vi "RSZVB Set Permanent Signal Generator State.vi"(6 "Generator Number (1)":i32=1, 7 "State (F: Off)":bool, 8 "error in (no error)":errorcluster {"code" format="%.0x"}, 9 "Port (1)":i32=1, 10 "Channel (1)":i32=1, 11 "VISA session":refnum<visa-resource-name>) -> (0 "error out":errorcluster {"code" format="%.0x"}, 3 "dup VISA session":refnum<visa-resource-name>)   [LabVIEW 2011]
doc: "This VI defines whether the external generator power is permanently on. \n\nNote(s):\n\n(1) This VI is available only on R&S ZVA instrument.\n\nRemote-control command(s):\nSOURce<Ch>:POWer<Pt>:GENerator<Gen>:PERManent[:STATe] <Boolean>"
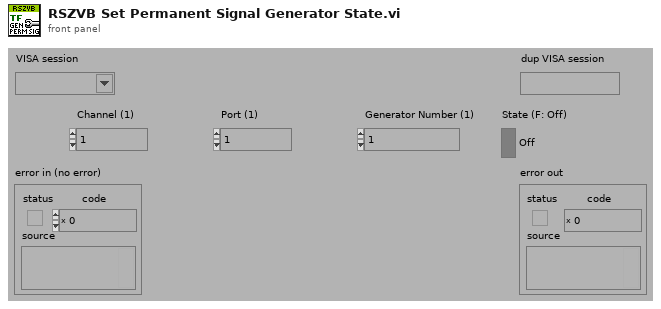
[diagram p1: front panel]
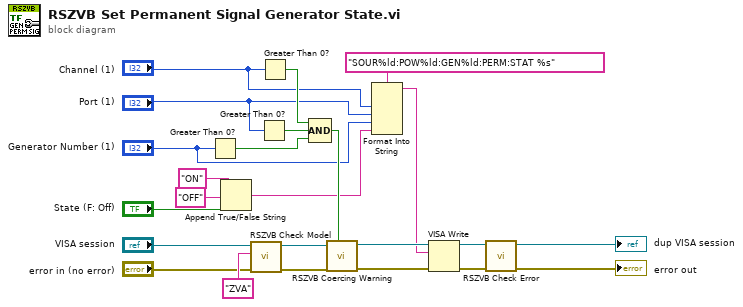
[diagram p0: block diagram]
diagram:
  n1 = Greater Than 0?(x="Generator Number (1)") -> (x > 0?=w8:bool)
  n2 = Append True/False String(1:"State (F: Off)", 2:"OFF", 3:"ON") -> (0:w7:string)  [unwired: 1 in]
  n3 = call "RSZVB Check Model.vi"("error in (no error)"="error in (no error)", "Model"="ZVA" ("Options"), "VISA session"="VISA session") -> ("error out"=w1:errorcluster, "dup VISA session"=w2:refnum<visa-resource-name>)  [unwired: 7 in]
  n4 = Greater Than 0?(x="Port (1)") -> (x > 0?=w14:bool)
  n5 = Greater Than 0?(x="Channel (1)") -> (x > 0?=w17:bool)
  n6 = Compound Arithmetic op=AND(w17, w14, w8) -> (w19:bool)
  n7 = call "RSZVB Coercing Warning.vi"("In Range?"=w19, "error in (no error)"=w1, "VISA session"=w2) -> ("error out"=w22:errorcluster, "dup VISA session"=w23:refnum<visa-resource-name>)  [unwired: 7 in]
  n8 = Format Into String(format string="SOUR%ld:POW%ld:GEN%ld:PERM:STAT %s", "Channel (1)", "Port (1)", "Generator Number (1)", w7) -> (resulting string=w18:string)  [unwired: 2 in, 1 out]
  n9 = VISA Write(VISA resource name=w23, write buffer=w18, error in (no error)=w22) -> (VISA resource name out=w20:refnum<visa-resource-name>, error out=w21:errorcluster)  [unwired: 1 out]
  n10 = call "RSZVB Check Error.vi"("error in (no error)"=w21, "VISA session"=w20) -> ("error out"=→"error out":errorcluster, "dup VISA session"=→"dup VISA session":refnum<visa-resource-name>)  [unwired: 8 in]
